vi "make_powerlog.vi"() -> ()   [LabVIEW 2025]
panel:
  out "Power":string
  out "Device":string
  in  "stop":bool
  out "Timestamp":string
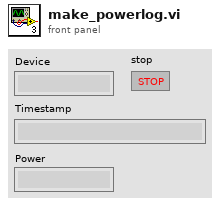
[diagram p1: front panel]
types:
  T1 = enum16{"open", "replace", "create", "open or create", "replace or create", "replace or create with confirmation"}
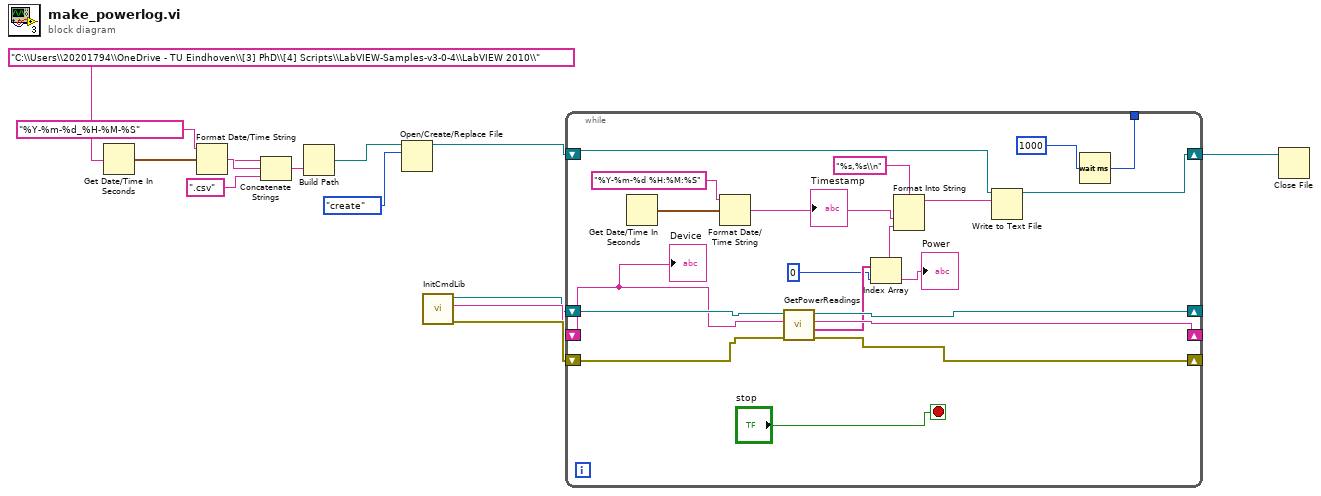
[diagram p0: block diagram]
diagram:
  n1 = Get Date/Time In Seconds() -> (seconds since 1Jan1904=w9:timestamp)
  n2 = Format Date/Time String(time format string (%c)="%Y-%m-%d_%H-%M-%S", seconds (now)=w9) -> (date/time string=w8:string)  [unwired: 1 in]
  n3 = Concatenate Strings("C:\\Users\\20201794\\OneDrive - TU Eindhoven\\[3] PhD\\[4] Scripts\\LabVIEW-Samples-v3-0-4\\LabVIEW 2010\\", w8, ".csv") -> (w5:string)
  n4 = Build Path(name or relative path=w5) -> (appended path=w4:path)  [unwired: 1 in]
  n5 = Open/Create/Replace File(file path (use dialog)=w4, operation (0:open)=T1."create") -> (refnum out=w2:refnum<file>)  [unwired: 4 in, 2 out]
  n6 = call "InitCmdLib.vi"() -> ("error out"=w13:errorcluster, "Device Key"=w12:string, "CmdLib"=w11:refnum<k24>)  [unwired: 9 in]
  n7 = while {
    shift-right: [w24] -> _
    shift-left: w11 -> [w29]
    shift-right: [w25] -> _
    shift-left: w12 -> [w28]
    shift-right: [w26] -> _
    shift-left: w13 -> [w27]
    shift-right: [w16] -> w1
    shift-left: w2 -> [w17]
    tunnel: [w14] -> _
    stop <- "stop" stop-if-true
    n8 = Get Date/Time In Seconds() -> (seconds since 1Jan1904=w32:timestamp)
    n9 = Format Date/Time String(time format string (%c)="%Y-%m-%d %H:%M:%S", seconds (now)=w32) -> (date/time string=w20:string)  [unwired: 1 in]
    "Timestamp" <- w20
    n10 = call "GetPowerReadings.vi"("error in"=w27, "Device Key In"=w28, "PM Cmds In"=w29) -> ("error out"=w26:errorcluster, "Power Readings"=w23:string[], "Device Key Out"=w25:string, "PM Cmds Out"=w24:refnum<k24>)  [unwired: 1 in]
    n11 = Index Array(array=w23, index=0) -> (element=w19:string)
    "Power" <- w19
    n12 = Format Into String(format string="%s,%s\\n", w20, w19) -> (resulting string=w18:string)  [unwired: 2 in, 1 out]
    n13 = Write to Text File(file (use dialog)=w17, text=w18) -> (refnum out=w16:refnum<file>)  [unwired: 2 in, 2 out]
    n14 = Wait (ms)(milliseconds to wait=1000) -> (millisecond timer value=w14:u32)
    "Device" <- w28
  }
  n15 = Close File(refnum=w1) -> ()  [unwired: 1 in, 2 out]
